vi "Write JSONMessage.vi"(8 "error in (no error)":errorcluster, 10 "wamplv.lvlib:JSONMessage.lvclass":refnum<class "JSONMessage.lvclass">, 11 "IJsonMessageHandler in":refnum<class "IJsonMessageHandler.lvclass">) -> (0 "error out":errorcluster, 3 "IJsonMessageHandler out":refnum<class "IJsonMessageHandler.lvclass">)   [LabVIEW 2020, in "wamplv.lvlib" / "IJsonMessageHandler.lvclass"]
uses:
  IJsonMessageHandler.lvclass
  IJsonMessageHandler.lvclass/IJsonMessageHandler.ctl
  SerialisedMessages/JSONMessage/JSONMessage.lvclass
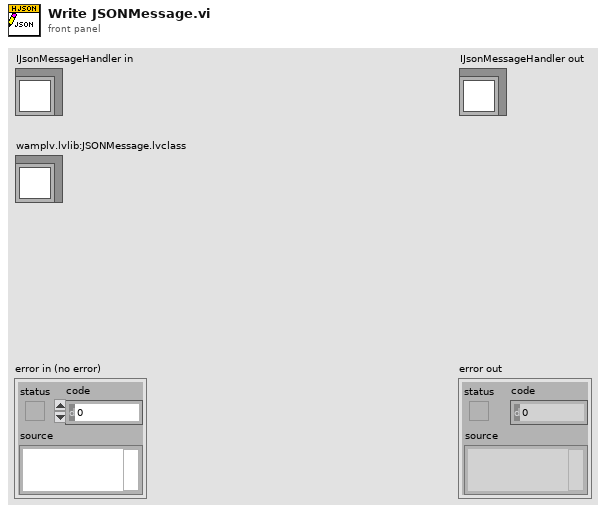
[diagram p1: front panel]
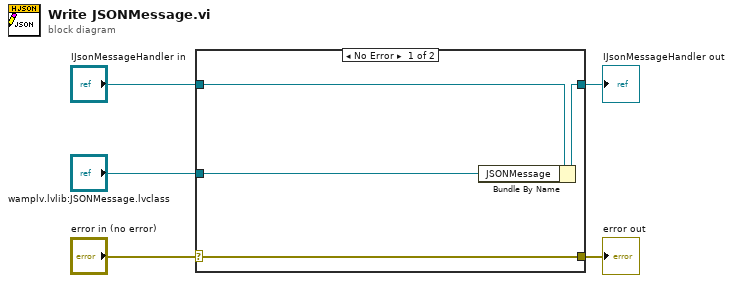
[diagram p0: block diagram]
diagram:
  n1 = case shown="No Error" "error in (no error)" {
    selector: "error in (no error)" -> [w9 w10]
    tunnel: [w9 w10] -> w4
    tunnel: [w7 w11] -> w2
    tunnel: "IJsonMessageHandler in" -> [w8 w11]
    tunnel: "wamplv.lvlib:JSONMessage.lvclass" -> [w6 _]
    frame No Error {
      n2 = Bundle By Name(cluster=w8, "JSONMessage"=w6) -> (w7:refnum<class "IJsonMessageHandler.lvclass">)
    }
    frame Error {
    }
  }
  "error out" <- w4
  "IJsonMessageHandler out" <- w2
